vi "Master.vi"   [LabVIEW 2015, in "Lego_Swerve_2015.lvrbt"]
uses:
  Lego_Swerve_2015.lvrbt
  <vilib>/NXT/Block Support/NXT_OutputPort.ctl
  <vilib>/NXT/Block Support/NXT_MessageMailbox.ctl
  <vilib>/NXT/Dual Mode Library/Motors/Rotation.vi
  <vilib>/NXT/Dual Mode Library/BT/BlueTooth_Write_String.vi
  <vilib>/NXT/Dual Mode Library/BT/BlueTooth_Write_String_c2.vi
  <vilib>/NXT/Dual Mode Library/BT/BlueTooth_Write_String_c3.vi
types:
  T1 = typedef "LVHSConnector.ctl" = refnum<class "BrickReference.lvclass">
  T2 = typedef "NXT_MessageMailbox.ctl" = u8
  T3 = typedef "NXT_OutputPort.ctl" = u8
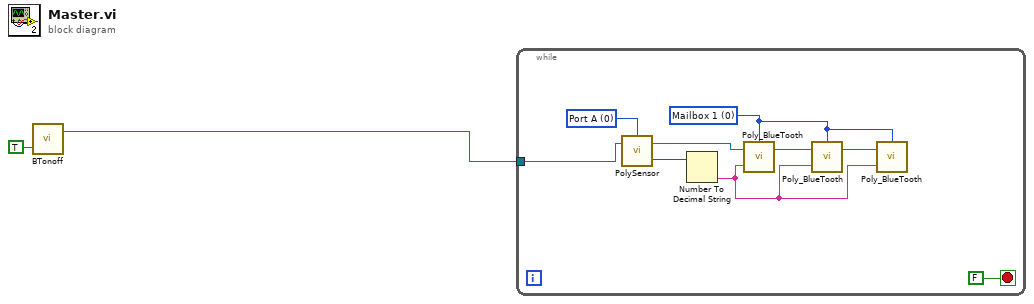
[diagram p0: block diagram]
diagram:
  n1 = call <vilib>:"BTonoff.vi"("On/Off"=TRUE) -> ("NXT/EV3"=w1:T1)  [unwired: 2 in, 1 out]
  n2 = while {
    tunnel: w1 -> [w8]
    stop <- FALSE stop-if-true
    w3 = T2 0 items=["Mailbox 1", "Mailbox 2", "Mailbox 3", "Mailbox 4", "Mailbox 5", "Mailbox 6", "Mailbox 7", "Mailbox 8", "Mailbox 9", "Mailbox 10"] ("Mailbox")
    w10 = T3 0 items=["Port A", "Port B", "Port C", "Port D"] ("Port (Port A)")
    n3 = call-poly <vilib>:"PolySensor.vi"("NXT/EV3"=w8, "Port (Port A)"=w10) -> ("Angle of Rotation"=w9:i32, "NXT/EV3"=w7:T1)  [unwired: 1 in]
    n4 = Number To Decimal String(number=w9) -> (decimal integer string=w4:string)  [unwired: 1 in]
    n5 = call-poly <vilib>:"Poly_BlueTooth.vi"("Message"=w4, "NXT/EV3"=w7, "Mailbox"=w3) -> ("NXT/EV3"=w6:T1)  [unwired: 1 in]
    n6 = call-poly <vilib>:"Poly_BlueTooth.vi"("Message"=w4, "NXT/EV3"=w6, "Mailbox"=w3) -> ("NXT/EV3"=w5:T1)  [unwired: 1 in]
    n7 = call-poly <vilib>:"Poly_BlueTooth.vi"("Message"=w4, "NXT/EV3"=w5, "Mailbox"=w3) -> ()  [unwired: 1 in, 1 out]
  }
